vi "Auto_Routine_StraightTwoPiece.vi"(8 "error in (no error)":errorcluster) -> (0 "error out":errorcluster)   [LabVIEW 2023]
uses:
  Shoulder/ShoulderGetSetpointEnum.ctl
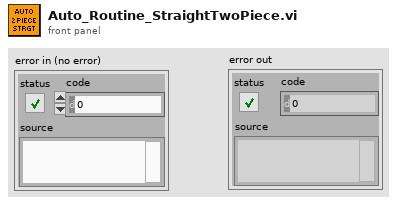
[diagram p1: front panel]
types:
  T1 = typedef "ShoulderGetSetpointEnum.ctl" = enum16{"ShoulderRest", "ShoulderSpeaker", "ShoulderAmp"}
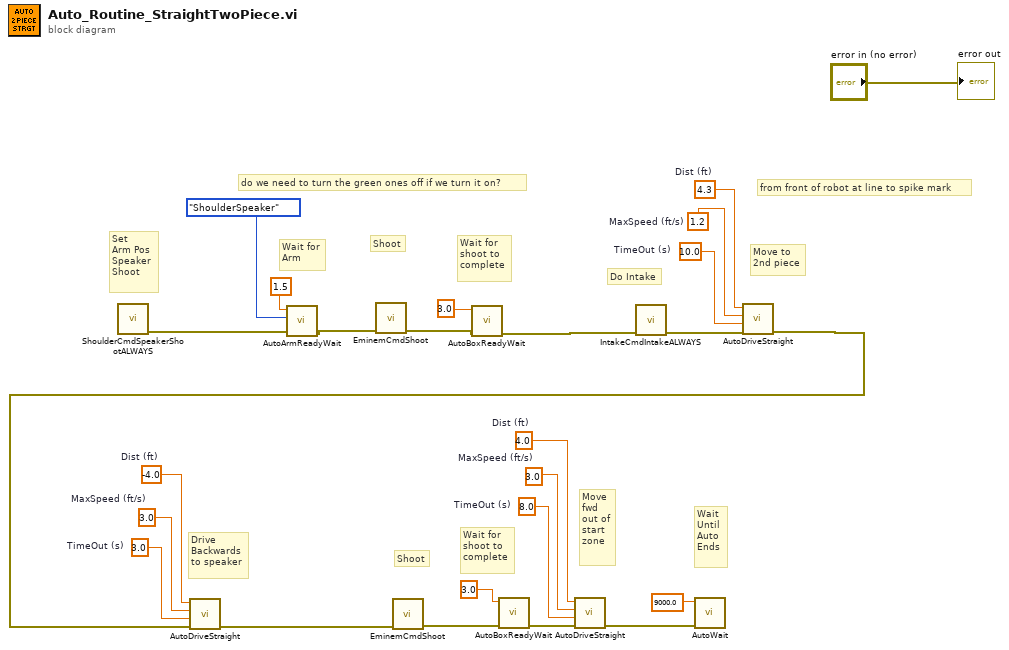
[diagram p0: block diagram]
diagram:
  w23 = 8.0  # TimeOut (s)
  w22 = 3.0  # MaxSpeed (ft/s)
  w21 = 4.0  # Dist (ft)
  w18 = 3.0  # TimeOut (s)
  w17 = 3.0  # MaxSpeed (ft/s)
  w16 = -4.0  # Dist (ft)
  w10 = 10.0  # TimeOut (s)
  w9 = 1.2  # MaxSpeed (ft/s)
  w8 = 4.3  # Dist (ft)
  # "Wait\nUntil\nAuto \nEnds"
  # "Move\nfwd\nout of\nstart\nzone"
  # "Wait for\nshoot to\ncomplete"
  # "Shoot"
  # "Drive\nBackwards\nto speaker"
  # "Do Intake"
  # "Move to \n2nd piece"
  # "Wait for\nshoot to\ncomplete"
  # "Shoot"
  # "Wait for\nArm"
  # "Set\nArm Pos\nSpeaker\nShoot"
  # "do we need to turn the green ones off if we turn it on?"
  # "from front of robot at line to spike mark"
  n1 = call "ShoulderCmdSpeakerShootALWAYS.vi"() -> ("error out"=w2:errorcluster)  [unwired: 11 in]
  n2 = call "AutoArmReadyWait.vi"("error in (no error)"=w2, "ArmSetpoints"=ShoulderGetSetpointEnum."ShoulderSpeaker", "TimeOut (s)"=1.5) -> ("error out"=w12:errorcluster)  [unwired: 8 in]
  n3 = call "EminemCmdShoot.vi"("error in (no error)"=w12) -> ("error out"=w14:errorcluster)  [unwired: 10 in]
  n4 = call "AutoBoxReadyWait.vi"("error in (no error)"=w14, "TimeOut (s)"=3.0) -> ("error out"=w4:errorcluster)  [unwired: 9 in]
  n5 = call "IntakeCmdIntakeALWAYS.vi"("error in (no error)"=w4) -> ("error out"=w3:errorcluster)  [unwired: 10 in]
  n6 = call "AutoDriveStraight.vi"("error in (no error)"=w3, "TimeOut (s)"=w10, "MaxSpeed (ft/s)"=w9, "Dist (ft)"=w8) -> ("error out"=w6:errorcluster)  [unwired: 7 in]
  n7 = call "AutoDriveStraight.vi"("error in (no error)"=w6, "TimeOut (s)"=w18, "MaxSpeed (ft/s)"=w17, "Dist (ft)"=w16) -> ("error out"=w1:errorcluster)  [unwired: 7 in]
  n8 = call "EminemCmdShoot.vi"("error in (no error)"=w1) -> ("error out"=w19:errorcluster)  [unwired: 10 in]
  n9 = call "AutoBoxReadyWait.vi"("error in (no error)"=w19, "TimeOut (s)"=3.0) -> ("error out"=w24:errorcluster)  [unwired: 9 in]
  n10 = call "AutoDriveStraight.vi"("error in (no error)"=w24, "TimeOut (s)"=w23, "MaxSpeed (ft/s)"=w22, "Dist (ft)"=w21) -> ("error out"=w25:errorcluster)  [unwired: 7 in]
  n11 = call "AutoWait.vi"("error in (no error)"=w25, "TimeOut (s)"=9000.0) -> ()  [unwired: 9 in, 1 out]
  "error out" <- "error in (no error)"
